vi "Get CustomDevice Reference.vi"(8 "error in":errorcluster, 11 "Item Ref in":u64 format="%.0x") -> (0 "error out":errorcluster, 2 "Custom Device":refnum<k24>, 3 "Item Ref out":u64 format="%.0x")   [LabVIEW 2026, in "Template Configuration.lvlib"]
uses:
  Template Configuration.lvlib
  NationalInstruments.VeriStand.SystemDefinitionAPI
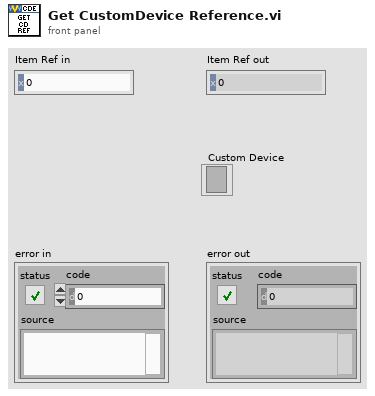
[diagram p1: front panel]
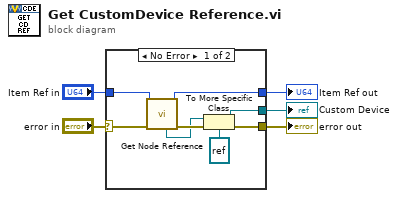
[diagram p0: block diagram]
diagram:
  n1 = case shown="No Error" "error in" {
    selector: "error in" -> [w13 w15]
    tunnel: [w7 w15] -> w4
    tunnel: "Item Ref in" -> [w11 w14]
    tunnel: [w12 w14] -> w2
    tunnel: [w6 _] -> w1
    frame No Error {
      n2 = call "Get Node Reference.vi"("error in"=w13, "Item Ref in"=w11) -> ("error out"=w10:errorcluster, "Item Ref out"=w12:u64, "Base Node"=w9:refnum<k24>)  [unwired: 6 in, 1 out]
      n3 = To More Specific Class(target class=refnum<k24> refnum ("IDToCustomDevice"), reference=w9, error in=w10) -> (specific class reference=w6:refnum<k24>, error out=w7:errorcluster)
    }
    frame Error {
    }
  }
  "error out" <- w4
  "Item Ref out" <- w2
  "Custom Device" <- w1
